vi "FTW-Example-Service-Core-Process.vi"(0 "FTW Actor Instance Configuration":string="{\n  \"Identity\": \"ActorName\",\n  \"InboxAddress\": \"inproc://*\",\n  \"PublisherAddress\": \"\",\n  \"LoggerAddress\": \"\",\n  \"DebugEnableInboxLogging\": false,\n  \"DebugEnableJobLogging\": false,\n  \"LauncherAddress\": \"\"\n}", 11 "error in":errorcluster) -> (15 "error out":errorcluster)   [LabVIEW 2013, in "FTW-Example-Service-Core.lvclass"]
uses:
  FTW-Example-Service-Core.lvclass
  source/actor/Instance/FTW-ActorInstance.lvclass/FTW-ActorInstance.ctl
  source/actor/JobSequencer/FTW-SEQ-Current.vi
  source/actor/Instance/FTW-ActorInstance.lvclass
  source/actor/Message/Request/FTW-Message-IncomingRequest.lvclass
  source/actor/Ether/FTW-Ether.lvclass
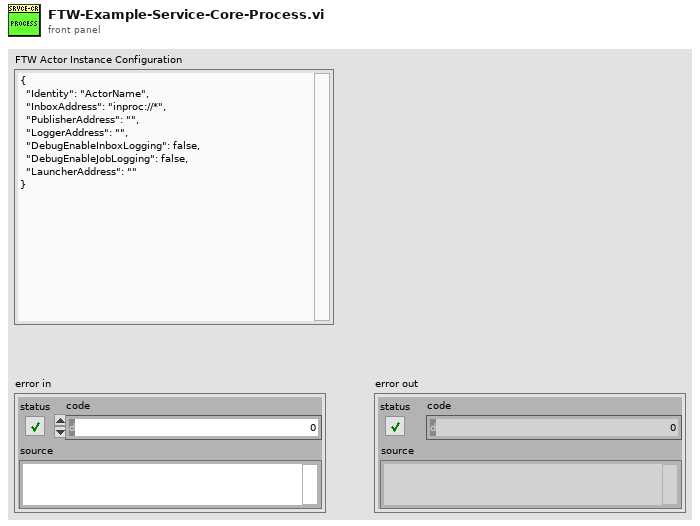
[diagram p1: front panel]
types:
  T1 = cluster{"Incoming Requests":refnum<event-registration>, "Additional Registration Types":refnum<event-registration>}
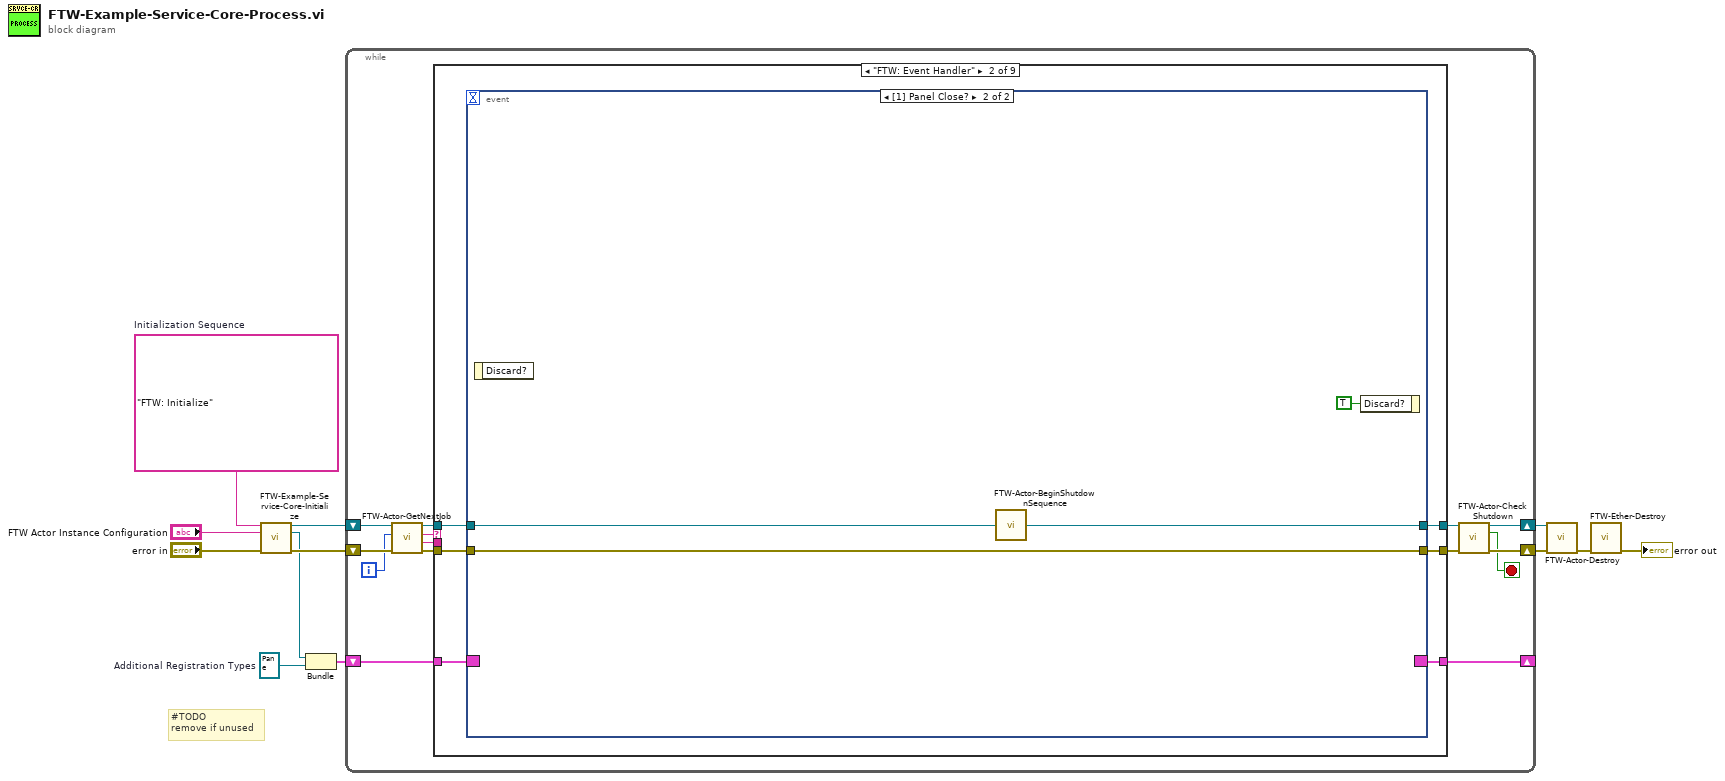
[diagram p0: block diagram]
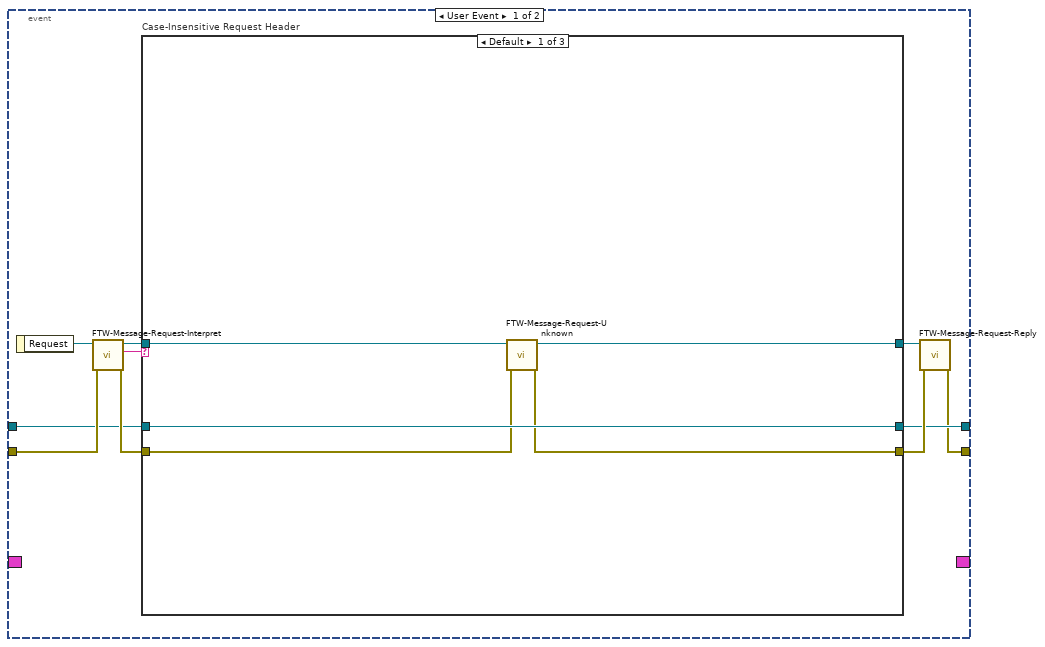
[diagram p3: hidden frame]
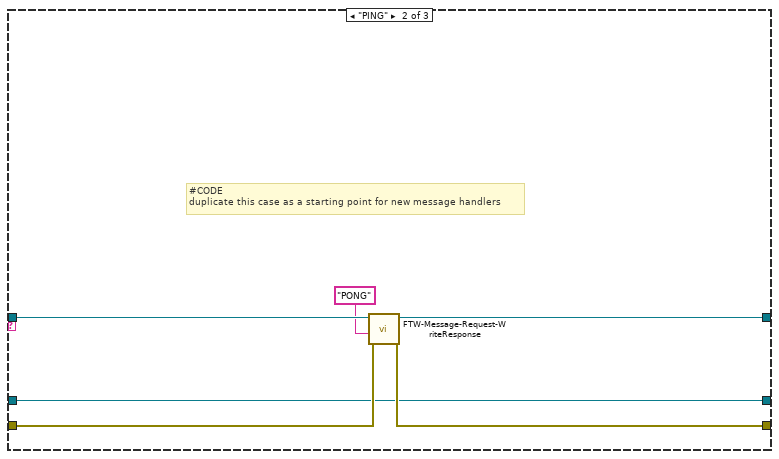
[diagram p4: hidden frame]
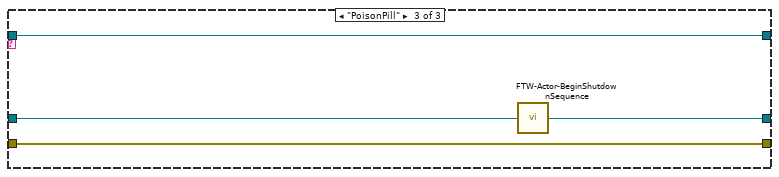
[diagram p5: hidden frame]
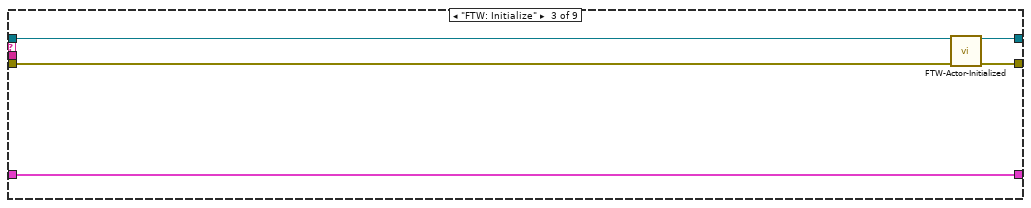
[diagram p6: hidden frame]
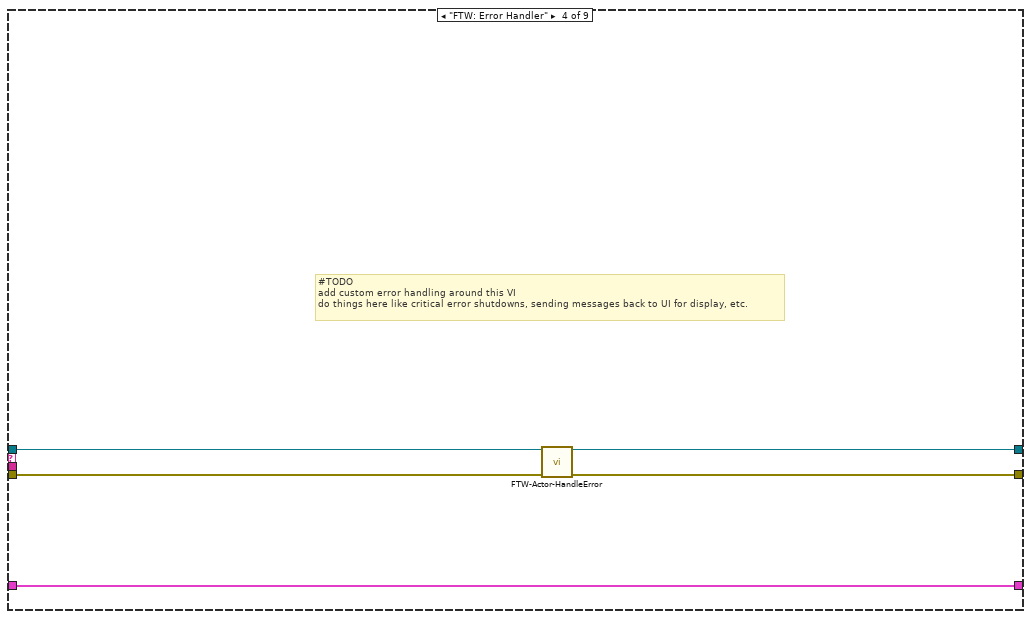
[diagram p7: hidden frame]
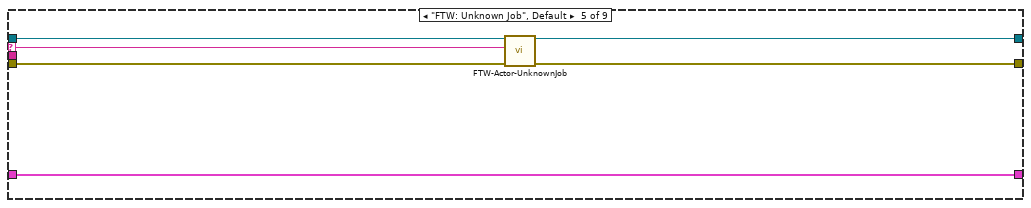
[diagram p8: hidden frame]
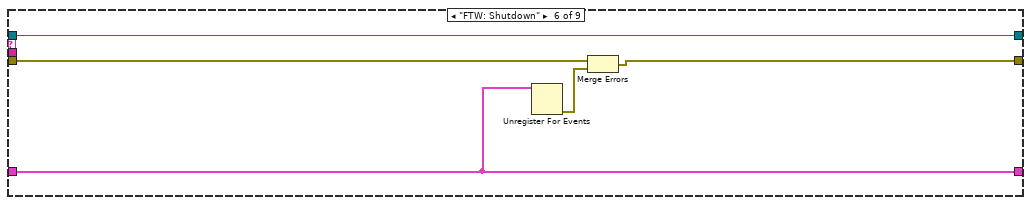
[diagram p9: hidden frame]
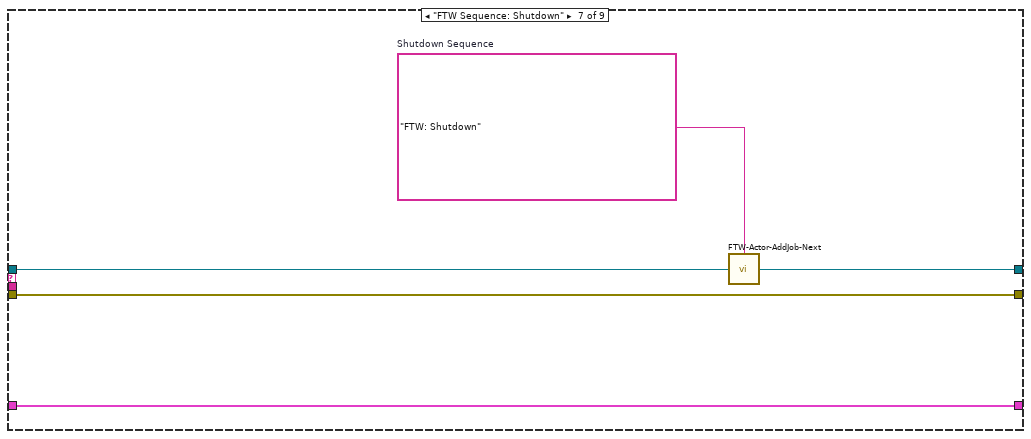
[diagram p10: hidden frame]
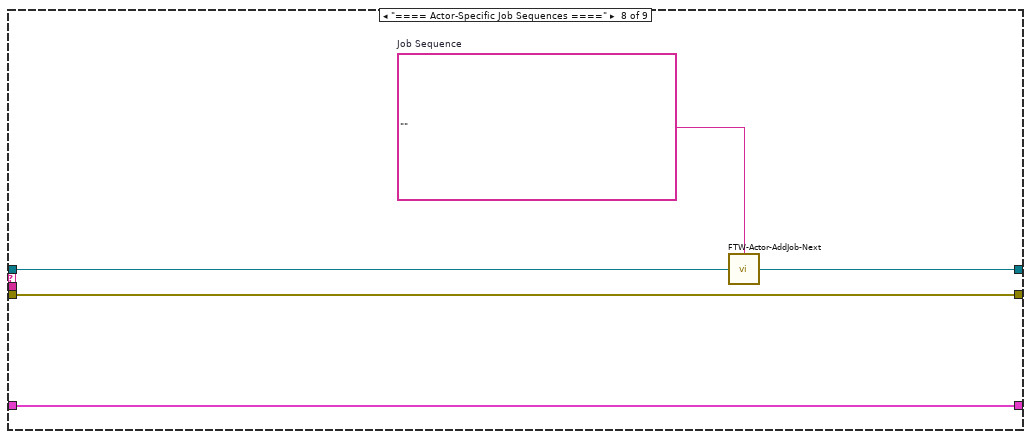
[diagram p11: hidden frame]
diagram:
  w6 = refnum<event-registration> refnum  # Additional Registration Types
  w7 = "FTW: Initialize"  # Initialization Sequence
  # "#TODO\nremove if unused"
  n1 = call "FTW-Example-Service-Core-Initialize.vi"("Initialization Sequence"=w7, "FTW Actor Instance Configuration"="FTW Actor Instance Configuration", "error in (no error)"="error in") -> ("Actor Template-Core out"=w12:refnum<class "FTW-Example-Service-Core.lvclass">, "Incoming Requests"=w4:refnum<event-registration>, "error out"=w8:errorcluster)  [unwired: 10 in]
  n2 = Bundle("Incoming Requests"=w4, "Additional Registration Types"=w6) -> (w5:T1)  [unwired: 1 in]
  n3 = while {
    shift-right: [w16] -> w10
    shift-left: w8 -> [w23]
    shift-right: [w13] -> _
    shift-left: w5 -> [w26]
    shift-right: [w18] -> w11
    shift-left: w12 -> [w25]
    i -> [w14]
    stop <- w15 stop-if-true
    n4 = call "FTW-Actor-GetNextJob.vi"("error in"=w23, "Jobs Performed"=w14, "FTW Actor Instance"=w25) -> ("error out"=w22:errorcluster, "Job Data"=w20:string, "Job Name"=w21:string, "FTW Actor Instance out"=w24:refnum<class "FTW-Example-Service-Core.lvclass">)  [unwired: 5 in]
    n5 = case shown="\"FTW: Event Handler\"" w21 {
      selector: w21 -> [_ _ _ _ w75 _ _ _ _]
      tunnel: [w28 w35 w65 w70 w78 w84 w89 w94 w98] -> w17
      tunnel: w22 -> [w28 w34 w68 w72 w79 w85 w89 w94 w98]
      tunnel: w26 -> [w29 w30 w69 w74 w80 w81 w90 w95 w97]
      tunnel: [w29 w33 w69 w74 w80 w81 w90 w95 w97] -> w13
      tunnel: w20 -> [_ _ _ _ _ _ _ _ _]
      tunnel: [w27 w32 w66 w71 w76 w82 w87 w92 w96] -> w19
      tunnel: w24 -> [w27 w31 w67 w73 w77 w82 w88 w93 w96]
      frame "==== Featherweight Framework Jobs ====" {
      }
      frame "FTW: Event Handler" {
        n6 = event shown="[1] Panel Close?" {
          selector: w30 -> [_ _]
          dyn-events: [_ _] -> w33
          timeout: _ -> [_ _]
          tunnel: [w38 w63] -> w35
          tunnel: w34 -> [w37 w63]
          tunnel: [w39 w61] -> w32
          tunnel: w31 -> [w36 w62]
          event User Event {
            n7 = event-data() -> ("Request"=w40:refnum<class "FTW-Message-IncomingRequest.lvclass">)  [unwired: 1 in]
            n8 = call "FTW-Message-Request-Interpret.vi"("error in"=w37, "FTW Incoming Request"=w40) -> ("error out"=w45:errorcluster, "Request Header"=w43:string, "FTW Incoming Request out"=w42:refnum<class "FTW-Message-IncomingRequest.lvclass">)  [unwired: 5 in, 2 out]
            n9 = case "Case-Insensitive Request Header" shown="Default" w43 {
              tunnel: [w48 w54 w59] -> w44
              tunnel: w45 -> [w49 w55 w59]
              tunnel: [w50 w53 w60] -> w39
              tunnel: w36 -> [w50 w53 w58]
              tunnel: w42 -> [w47 w56 w57]
              tunnel: [w46 w52 w57] -> w41
              frame Default {
                n10 = call "FTW-Message-Request-Unknown.vi"("error in"=w49, "FTW Incoming Request"=w47) -> ("error out"=w48:errorcluster, "FTW Incoming Request Out"=w46:refnum<class "FTW-Message-IncomingRequest.lvclass">)  [unwired: 8 in]
              }
              frame "PING" {
                # "#CODE\nduplicate this case as a starting point for new message handlers"
                n11 = call "FTW-Message-Request-WriteResponse.vi"("error in"=w55, "Response Body"="PONG" ("Response Header"), "FTW Incoming Request"=w56) -> ("error out"=w54:errorcluster, "FTW Incoming Request out"=w52:refnum<class "FTW-Message-IncomingRequest.lvclass">)  [unwired: 7 in]
              }
              frame "PoisonPill" {
                n12 = call "FTW-Actor-BeginShutdownSequence.vi"("FTW Actor Instance"=w58) -> ("FTW Actor Instance out"=w60:refnum<class "FTW-Example-Service-Core.lvclass">)  [unwired: 3 in]
              }
            }
            n13 = call "FTW-Message-Request-Reply.vi"("FTW: Reply Error"=w44, "FTW Incoming Request"=w41) -> ("error out"=w38:errorcluster)  [unwired: 8 in, 1 out]
          }
          event Panel Close? {
            n14 = event-data() -> ()  [unwired: 1 in, 1 out]
            n15 = call "FTW-Actor-BeginShutdownSequence.vi"("FTW Actor Instance"=w62) -> ("FTW Actor Instance out"=w61:refnum<class "FTW-Example-Service-Core.lvclass">)  [unwired: 3 in]
            n16 = event-data("Discard?"=TRUE) -> ()  [unwired: 1 in, 1 out]
          }
        }
      }
      frame "FTW: Initialize" {
        n17 = call-dynamic "FTW-Actor-Initialized.vi"("FTW Actor Instance"=w67, "error in"=w68) -> ("FTW Actor Instance out"=w66:refnum<class "FTW-Example-Service-Core.lvclass">, "error out"=w65:errorcluster)  [unwired: 12 in]
      }
      frame "FTW: Error Handler" {
        # "#TODO\nadd custom error handling around this VI\ndo things here like critical error shutdowns, sending messages back to UI for display, etc."
        n18 = call-dynamic "FTW-Actor-HandleError.vi"("FTW Actor Instance"=w73, "error in"=w72) -> ("FTW Actor Instance out"=w71:refnum<class "FTW-Example-Service-Core.lvclass">, "error out"=w70:errorcluster)  [unwired: 10 in, 2 out]
      }
      frame "FTW: Unknown Job", Default {
        n19 = call-dynamic "FTW-Actor-UnknownJob.vi"("FTW Actor Instance"=w77, "Unknown Job"=w75, "error in"=w79) -> ("FTW Actor Instance out"=w76:refnum<class "FTW-Example-Service-Core.lvclass">, "error out"=w78:errorcluster)  [unwired: 11 in]
      }
      frame "FTW: Shutdown" {
        n20 = Unregister For Events(event registration refnum=w81) -> (error out=w83:errorcluster)  [unwired: 1 in]
        n21 = Merge Errors(w85, w83) -> (w84:errorcluster)
      }
      frame "FTW Sequence: Shutdown" {
        w86 = "FTW: Shutdown"  # Shutdown Sequence
        n22 = call "FTW-Actor-AddJob-Next.vi"("Add Next in Job Queue"=w86, "FTW Actor Instance"=w88) -> ("FTW Actor Instance out"=w87:refnum<class "FTW-Example-Service-Core.lvclass">)  [unwired: 2 in]
      }
      frame "==== Actor-Specific Job Sequences ====" {
        w91 = ""  # Job Sequence
        n23 = call "FTW-Actor-AddJob-Next.vi"("Add Next in Job Queue"=w91, "FTW Actor Instance"=w93) -> ("FTW Actor Instance out"=w92:refnum<class "FTW-Example-Service-Core.lvclass">)  [unwired: 2 in]
      }
      frame "==== Actor-Specific Jobs ====" {
      }
    }
    n24 = call "FTW-Actor-CheckShutdown.vi"("FTW Actor Instance"=w19, "error in"=w17) -> ("FTW Actor Instance out"=w18:refnum<class "FTW-Example-Service-Core.lvclass">, "Shutdown?"=w15:bool, "error out"=w16:errorcluster)  [unwired: 11 in]
  }
  n25 = call-dynamic "FTW-Actor-Destroy.vi"("FTW Actor Instance"=w11, "error in"=w10) -> ("error out"=w9:errorcluster)  [unwired: 13 in]
  n26 = call "FTW-Ether-Destroy.vi"("error in"=w9) -> ("error out"=→"error out":errorcluster)  [unwired: 14 in]
